vi "BestFitLine.vi"(6 "Function":enum16{"End", "Start"}(ring)=enum."Start", 8 "Found Line":i32, 9 "Intersect Point":cluster{"X":dbl, "Y":dbl, "Z":dbl}, 10 "Tested Line":i32, 11 "All Lines":T2) -> (1 "Connection out":i32, 3 "Line out":i32)   [LabVIEW 2014]
uses:
  Libraries/Map Data Folder/All-Lines.ctl
  Libraries/Map Data Folder/LineCluster.ctl
  Libraries/Map Data Folder/LineConnection.ctl
  <vilib>/Analysis/6fits.llb/Curve Fitting Criteria.ctl
  <vilib>/Analysis/NI_AALPro.lvlib
  Libraries/Map Data Folder/Map Data.lvlib
panel:
  in  "milliseconds to wait":u32
  in  "method":T1 items=["Least Square", "Least Absolute Residual", "Bisquare"]
  out "Better Fit":string
  out "Found Line residue":dbl
  out "Tested Line residue":dbl
  out "XY Graph":cluster{dbl[], "Best Linear Fit":dbl[]}[](graph)
  in  "Sub length":i32=20
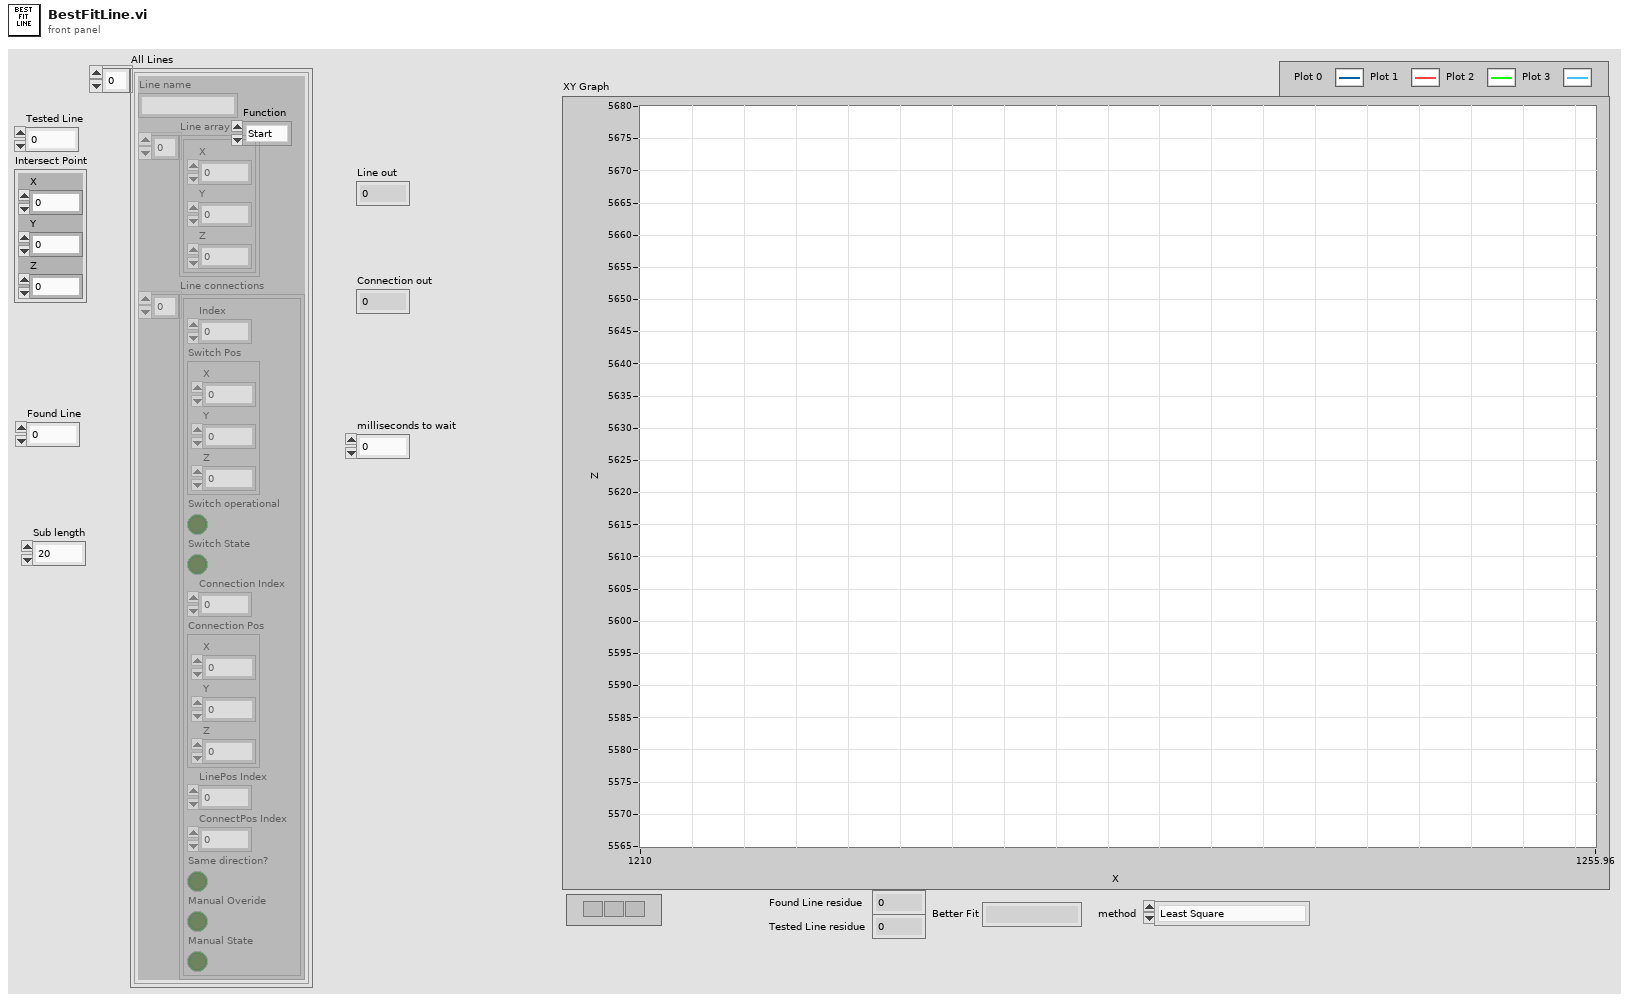
[diagram p1: front panel]
types:
  T1 = typedef "NI_AALPro.lvlib/Curve Fitting Criteria.ctl" = u16
  T2 = typedef "Map Data.lvlib/All-Lines.ctl" = T3[]
  T3 = typedef "Map Data.lvlib/LineCluster.ctl" = cluster{"Line name":string, "Line array":cluster{"X":dbl, "Y":dbl, "Z":dbl}[], "Line connections":T4[]}
  T4 = typedef "Map Data.lvlib/LineConnection.ctl" = cluster{"Index":i32, "Switch Pos":cluster{"X":dbl, "Y":dbl, "Z":dbl}, "Switch operational":bool, "Switch State":bool, "Connection Index":i32, "Connection Pos":cluster{"X":dbl, "Y":dbl, "Z":dbl}, "LinePos Index":i32, "ConnectPos Index":i32, "Same direction?":bool, "Manual Overide":bool, "Manual State":bool}
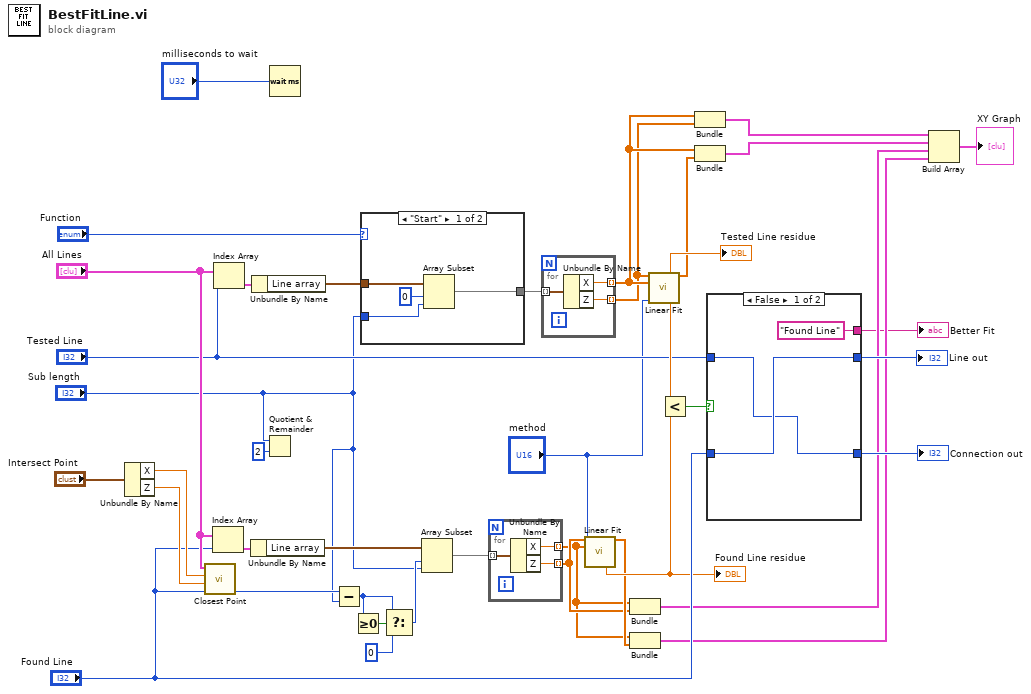
[diagram p0: block diagram]
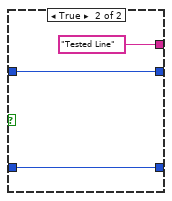
[diagram p2: hidden frame]
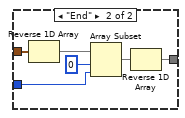
[diagram p3: hidden frame]
diagram:
  n1 = Unbundle By Name("Intersect Point") -> ("X"=w38:dbl, "Z"=w37:dbl)
  n2 = call "Closest Point.vi"("index"="Found Line", "Y in"=w37, "X in"=w38, "All Lines"="All Lines") -> ("Index on Line"=w29:i32)  [unwired: 5 in, 2 out]
  n3 = Index Array(array="All Lines", index="Found Line") -> (element=w36:T3)
  n4 = Index Array(array="All Lines", index="Tested Line") -> (element=w35:T3)
  n5 = Unbundle By Name(w36) -> ("Line array"=w30:cluster{"X":dbl, "Y":dbl, "Z":dbl}[])
  n6 = Unbundle By Name(w35) -> ("Line array"=w32:cluster{"X":dbl, "Y":dbl, "Z":dbl}[])
  n7 = Quotient & Remainder(x="Sub length", y=2) -> ()  [unwired: 2 out]
  n8 = Wait (ms)(milliseconds to wait="milliseconds to wait") -> ()  [unwired: 1 out]
  n9 = Subtract(x=w29, y="Sub length") -> (x-y=w25:i32)
  n10 = Greater Or Equal To 0?(x=w25) -> (x >= 0?=w28:bool)
  n11 = case shown="\"Start\"" "Function" {
    tunnel: w32 -> [w43 w48]
    tunnel: [w41 w45] -> w23
    tunnel: "Sub length" -> [w40 w44]
    frame "Start" {
      n12 = Array Subset(array=w43, index=0, length=w40) -> (w41:cluster{"X":dbl, "Y":dbl, "Z":dbl}[])
    }
    frame "End" {
      n13 = Reverse 1D Array(array=w48) -> (reversed array=w47:cluster{"X":dbl, "Y":dbl, "Z":dbl}[])
      n14 = Array Subset(array=w47, index=0, length=w44) -> (w46:cluster{"X":dbl, "Y":dbl, "Z":dbl}[])
      n15 = Reverse 1D Array(array=w46) -> (reversed array=w45:cluster{"X":dbl, "Y":dbl, "Z":dbl}[])
    }
  }
  n16 = Select(t=w25, s=w28, f=0 ("x-y")) -> (s? t:f=w26:i32)
  n17 = Array Subset(array=w30, index=w26, length="Sub length") -> (w24:cluster{"X":dbl, "Y":dbl, "Z":dbl}[])
  n18 = for {
    tunnel: w24 -> [w52] mode=indexing
    tunnel: [w51] -> w3 mode=indexing
    tunnel: [w50] -> w4 mode=indexing
    n19 = Unbundle By Name(w52) -> ("X"=w51:dbl, "Z"=w50:dbl)
  }
  n20 = for {
    tunnel: w23 -> [w55] mode=indexing
    tunnel: [w54] -> w16 mode=indexing
    tunnel: [w53] -> w5 mode=indexing
    n21 = Unbundle By Name(w55) -> ("X"=w54:dbl, "Z"=w53:dbl)
  }
  n22 = call <vilib>:"Linear Fit.vi"("Y"=w4, "X"=w3, "method"="method") -> ("Best Linear Fit"=w7:dbl[], "residue"=w10:dbl)  [unwired: 8 in, 3 out]
  "Found Line residue" <- w10
  n23 = Bundle(w3, w4) -> (w12:cluster{dbl[], dbl[]})  [unwired: 1 in]
  n24 = Bundle(w3, "Best Linear Fit"=w7) -> (w11:cluster{dbl[], "Best Linear Fit":dbl[]})  [unwired: 1 in]
  n25 = call <vilib>:"Linear Fit.vi"("Y"=w5, "X"=w16, "method"="method") -> ("Best Linear Fit"=w6:dbl[], "residue"=w22:dbl)  [unwired: 8 in, 3 out]
  "Tested Line residue" <- w22
  n26 = Less?(x=w22, y=w10) -> (x < y?=w21:bool)
  n27 = Bundle(w16, w5) -> (w15:cluster{dbl[], dbl[]})  [unwired: 1 in]
  n28 = Bundle(w16, "Best Linear Fit"=w6) -> (w14:cluster{dbl[], "Best Linear Fit":dbl[]})  [unwired: 1 in]
  n29 = case shown="False" w21 {
    tunnel: "Tested Line" -> [w57 w61]
    tunnel: "Found Line" -> [w58 w60]
    tunnel: [w58 w61] -> w18
    tunnel: [w57 w60] -> w17
    tunnel: ["Found Line" "Tested Line"] -> w9
    frame False {
    }
    frame True {
    }
  }
  "Line out" <- w18
  "Connection out" <- w17
  "Better Fit" <- w9
  n30 = Build Array(w15, w14, w12, w11) -> (→"XY Graph":cluster{dbl[], "Best Linear Fit":dbl[]}[])
